vi "RxPkt - Export Channel Configuration.vi"(8 "error in (no error)":errorcluster, 11 "Packet Ref in":T1 format="%.0x") -> (0 "error out":errorcluster, 3 "Packet Ref out":T1 format="%.0x")   [LabVIEW 2023, in "UDP-Custom-Device System Explorer.lvlib"]
uses:
  UDP-Custom-Device System Explorer.lvlib
  <vilib>/NI VeriStand/Custom Device API/Custom Device Item Ref.ctl
  Types/Channel Configuration/Channel Config File Data.ctl
  <vilib>/NI VeriStand/Custom Device API/Custom Device API.lvlib
  Shared/UDP-Custom-Device Shared.lvlib
  Property Accessors/Rx Channel Section Accessors.lvlib
  Property Accessors/Rx Channel Accessors.lvlib
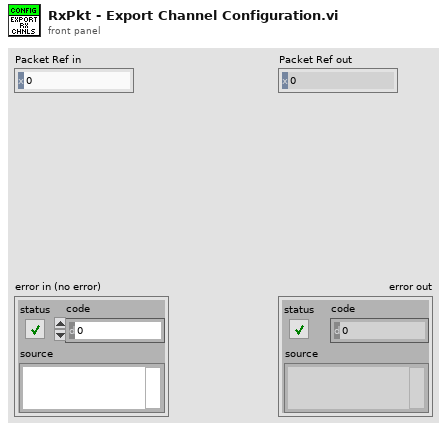
[diagram p1: front panel]
types:
  T1 = typedef "Custom Device API.lvlib/Custom Device Item Ref.ctl" = u64
  T2 = typedef "UDP-Custom-Device System Explorer.lvlib/Channel Config File Data.ctl" = cluster{"Signal Names":string[], "Channel Names":string[], "Channel Data Types":string[], "Channel Descriptions":string[]}
  T3 = typedef "Custom Device API.lvlib/Custom Device Item Info.ctl" = cluster{"Name":string, "Is Channel":bool, "GUID":string, "Is Waveform":bool}
  T4 = typedef "UDP-Custom-Device Shared.lvlib/Shared - Channel Data Type.ctl" = enum16{"Boolean", "Single", "Double", "I8", "I16", "I32", "I64", "U8", "U16", "U32", "U64"}
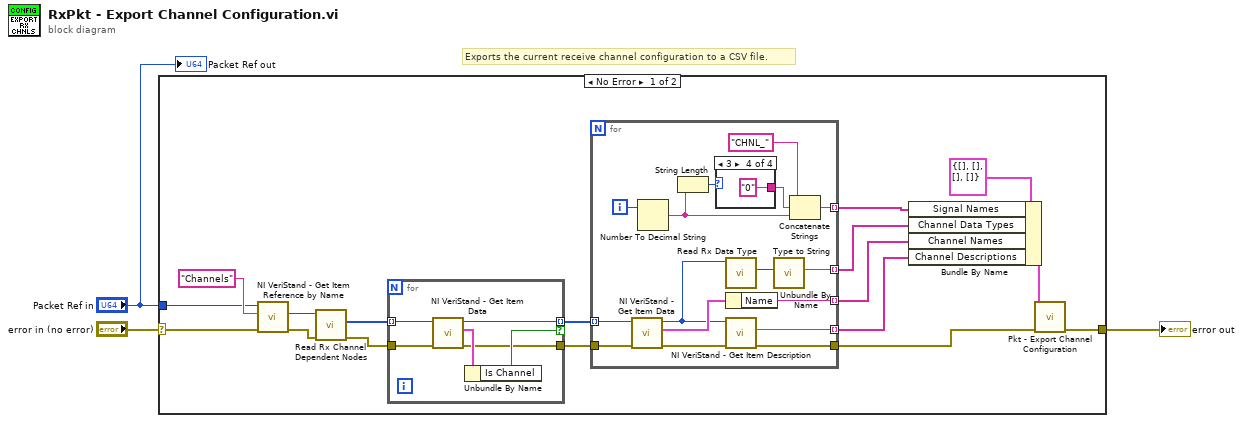
[diagram p0: block diagram]
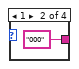
[diagram p3: hidden frame]
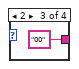
[diagram p4: hidden frame]
diagram:
  # "Exports the current receive channel configuration to a CSV file."
  n1 = case shown="No Error" "error in (no error)" {
    selector: "error in (no error)" -> [w8 w46]
    tunnel: "Packet Ref in" -> [w9 _]
    tunnel: [w19 w46] -> w2
    frame No Error {
      n2 = call <vilib>:"NI VeriStand - Get Item Reference by Name.vi"("error in (no error)"=w8, "Item Name"="Channels" ("Section Name"), "Parent Ref in"=w9) -> ("error out"=w10:errorcluster, "Item Ref"=w11:T1)  [unwired: 5 in, 2 out]
      n3 = call "Read Rx Channel Dependent Nodes.vi"("error in (no error)"=w10, "Node Ptr"=w11) -> ("error out"=w6:errorcluster, "Dependent Node Refs"=w7:T1[])  [unwired: 7 in, 1 out]
      n4 = for {
        tunnel: w7 -> [w25] mode=indexing
        tunnel: w6 -> [w24]
        tunnel: [w23] -> w5 mode=indexing if=w22
        tunnel: [w21] -> w4
        n5 = call <vilib>:"NI VeriStand - Get Item Data.vi"("error in (no error)"=w24, "Item Ref in"=w25) -> ("error out"=w21:errorcluster, "Item Info"=w26:T3, "Item Ref out"=w23:T1)  [unwired: 6 in, 1 out]
        n6 = Unbundle By Name(w26) -> ("Is Channel"=w22:bool)
      }
      n7 = for {
        tunnel: w4 -> [w32]
        tunnel: w5 -> [w30] mode=indexing
        tunnel: [w42] -> w14 mode=indexing
        tunnel: [w41] -> w20
        tunnel: [w34] -> w15 mode=indexing
        tunnel: [w38] -> w17 mode=indexing
        tunnel: [w35] -> w16 mode=indexing
        i -> [w40]
        n8 = call <vilib>:"NI VeriStand - Get Item Data.vi"("error in (no error)"=w32, "Item Ref in"=w30) -> ("error out"=w33:errorcluster, "Item Info"=w36:T3, "Item Ref out"=w31:T1)  [unwired: 6 in, 1 out]
        n9 = Number To Decimal String(number=w40) -> (decimal integer string=w27:string)  [unwired: 1 in]
        n10 = String Length(string=w27) -> (length=w29:i32)
        n11 = case shown="3" w29 {
          tunnel: [_ "000" ("Description") "00" ("Description") "0" ("Description")] -> w28
          frame Default {
          }
          frame 1 {
          }
          frame 2 {
          }
          frame 3 {
          }
        }
        n12 = call "Read Rx Data Type.vi"("Node Ptr"=w31) -> ("Data Type"=w37:T4)  [unwired: 8 in, 2 out]
        n13 = Unbundle By Name(w36) -> ("Name"=w34:string)
        n14 = call <vilib>:"NI VeriStand - Get Item Description.vi"("error in (no error)"=w33, "Item Ref in"=w31) -> ("error out"=w41:errorcluster, "Description"=w42:string)  [unwired: 6 in, 2 out]
        n15 = call "Type to String.vi"("Data Type"=w37) -> ("String Type"=w35:string)  [unwired: 10 in]
        n16 = Concatenate Strings("CHNL_" ("Description"), w28, w27) -> (w38:string)
      }
      n17 = Bundle By Name(cluster=T2 {"Signal Names"=[], "Channel Names"=[], "Channel Data Types"=[], "Channel Descriptions"=[]} ("Channel Config Data"), "Signal Names"=w17, "Channel Data Types"=w16, "Channel Names"=w15, "Channel Descriptions"=w14) -> (w13:T2)
      n18 = call "Pkt - Export Channel Configuration.vi"("error in (no error)"=w20, "Channel Config Data"=w13) -> ("error out"=w19:errorcluster)  [unwired: 9 in]
    }
    frame Error {
    }
  }
  "error out" <- w2
  "Packet Ref out" <- "Packet Ref in"
